vi "TestThorlabs.vi"() -> ()   [LabVIEW 2018]
uses:
  Mode.ctl
  Thorlabs_SC10.lvlib
panel:
  in  "Mode":T1
  out "error out":errorcluster
  in  "stop":bool
  in  "Toggle Shutter":bool
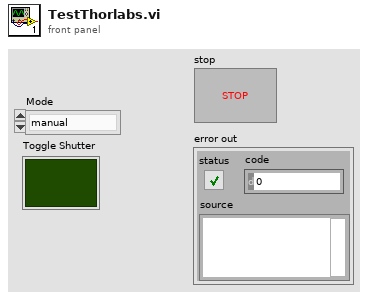
[diagram p1: front panel]
types:
  T1 = typedef "Thorlabs_SC10.lvlib/Mode.ctl" = enum16{"manual", "auto", "single", "repeat", "external gate"}
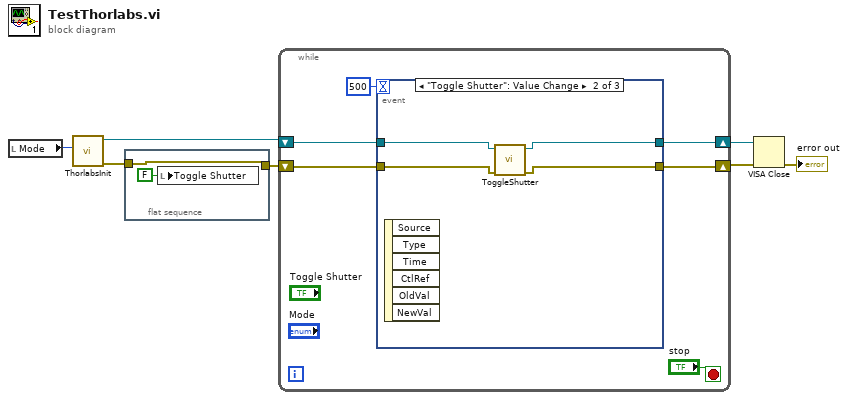
[diagram p0: block diagram]
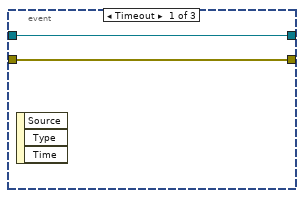
[diagram p2: hidden frame]
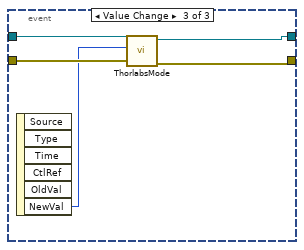
[diagram p3: hidden frame]
diagram:
  n1 = local read "Mode"() -> (w1:T1)
  n2 = call "ThorlabsInit.vi"("Shutter Mode"=w1) -> ("error out"=w4:errorcluster, "VISA resource name out"=w2:refnum<visa-resource-name>)  [unwired: 9 in]
  n3 = flat-sequence {
    tunnel: w4 -> [w8]
    tunnel: [w8] -> w3
    frame #0 {
      n4 = local write "Toggle Shutter"(FALSE ("Toggle Shutter")) -> ()
    }
  }
  n5 = while {
    shift-right: [w14] -> w6
    shift-left: w3 -> [w10]
    shift-right: [w15] -> w7
    shift-left: w2 -> [w11]
    stop <- "stop" stop-if-true
    n6 = event shown="[1] \"Toggle Shutter\": Value Change" {
      selector: _ -> [_ _ _]
      dyn-events: _ -> [_ _ _]
      timeout: 500 -> [_ _ _]
      tunnel: w11 -> [w17 w20 w23]
      tunnel: [w17 w19 w22] -> w15
      tunnel: [w16 w18 w25] -> w14
      tunnel: w10 -> [w16 w21 w26]
      event Timeout {
        n7 = event-data() -> ()  [unwired: 1 in, 3 out]
      }
      event "Toggle Shutter": Value Change {
        n8 = event-data() -> ()  [unwired: 1 in, 6 out]
        n9 = call "ToggleShutter.vi"("error in"=w21, "VISA resource name"=w20) -> ("error out"=w18:errorcluster, "VISA resource name out"=w19:refnum<visa-resource-name>)  [unwired: 8 in]
      }
      event Value Change {
        n10 = event-data() -> ("NewVal"=w24:T1)  [unwired: 1 in, 5 out]
        n11 = call "ThorlabsMode.vi"("error in"=w26, "Mode"=w24, "VISA resource name"=w23) -> ("error out"=w25:errorcluster, "VISA resource name out"=w22:refnum<visa-resource-name>)  [unwired: 7 in]
      }
    }
  }
  n12 = VISA Close(VISA resource name=w7, error in (no error)=w6) -> (error out=→"error out":errorcluster)
